vi "Perform Action.vi"(7 "IPerform Action":refnum<class "Instrument.lvclass">, 8 "error in":errorcluster, 10 "Input":variant, 11 "Perform Action Strategy in":refnum<class "Perform Action Strategy.lvclass">) -> (0 "error out":errorcluster, 2 "Output":variant, 3 "Perform Action Strategy out":refnum<class "Perform Action Strategy.lvclass">)   [LabVIEW 2023, in "HAL.lvlib" / "Perform Action Strategy.lvclass"]
uses:
  Perform Action Strategy.lvclass
  Instrument/Instrument.lvclass
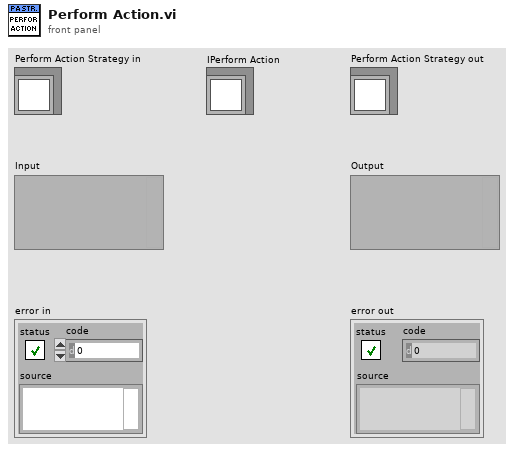
[diagram p1: front panel]
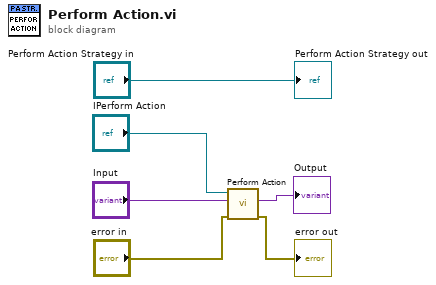
[diagram p0: block diagram]
diagram:
  n1 = call "Perform Action.vi"("Error In"="error in", "Input"="Input", "reference in"="IPerform Action") -> ("Error Out"=→"error out":errorcluster, "Output"=→"Output":variant)  [unwired: 6 in, 1 out]
  "Perform Action Strategy out" <- "Perform Action Strategy in"
